vi "Code_rijden.vi"() -> ()   [LabVIEW 2014]
uses:
  <vilib>/LabVIEW Interface for Arduino/Type Defs/Board Type.ctl
  <vilib>/LabVIEW Interface for Arduino/Type Defs/Connection Type.ctl
  <vilib>/LabVIEW Interface for Arduino/LabVIEW Interface for Arduino.lvlib
panel:
  in  "Value (0)":u8
  in  "Banden Rechts":u8
  in  "Banden Links":u8
  in  "Achter Rechts":u8(slide) scale=0.0..255.0
  in  "Achter Links":u8(slide) scale=0.0..255.0
  in  "Voor Rechts":u8(slide) scale=0.0..255.0
  in  "Voor Links":u8(slide) scale=0.0..255.0
  in  "STOP":bool
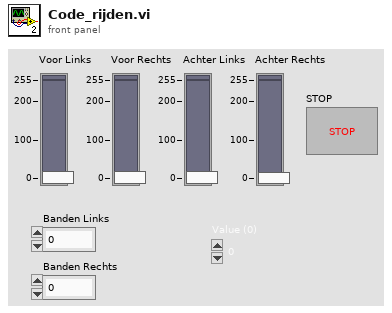
[diagram p1: front panel]
types:
  T1 = typedef "LabVIEW Interface for Arduino.lvlib/Connection Type.ctl" = enum8{"USB / Serial", "XBEE", "BlueSmirf (Bluetooth)"}
  T2 = typedef "LabVIEW Interface for Arduino.lvlib/Board Type.ctl" = enum16{"Uno", "Dimuelanove w/Atmega 328", "Mega 2560"}
  T3 = typedef "LabVIEW Interface for Arduino.lvlib/Arduino Resource.ctl" = cluster{"VISA resource":refnum<visa-resource-name>, "Board Type":T2, "Connection Type":enum8{"USB / Serial"}, "Bytes Per Packet (15)":u8}
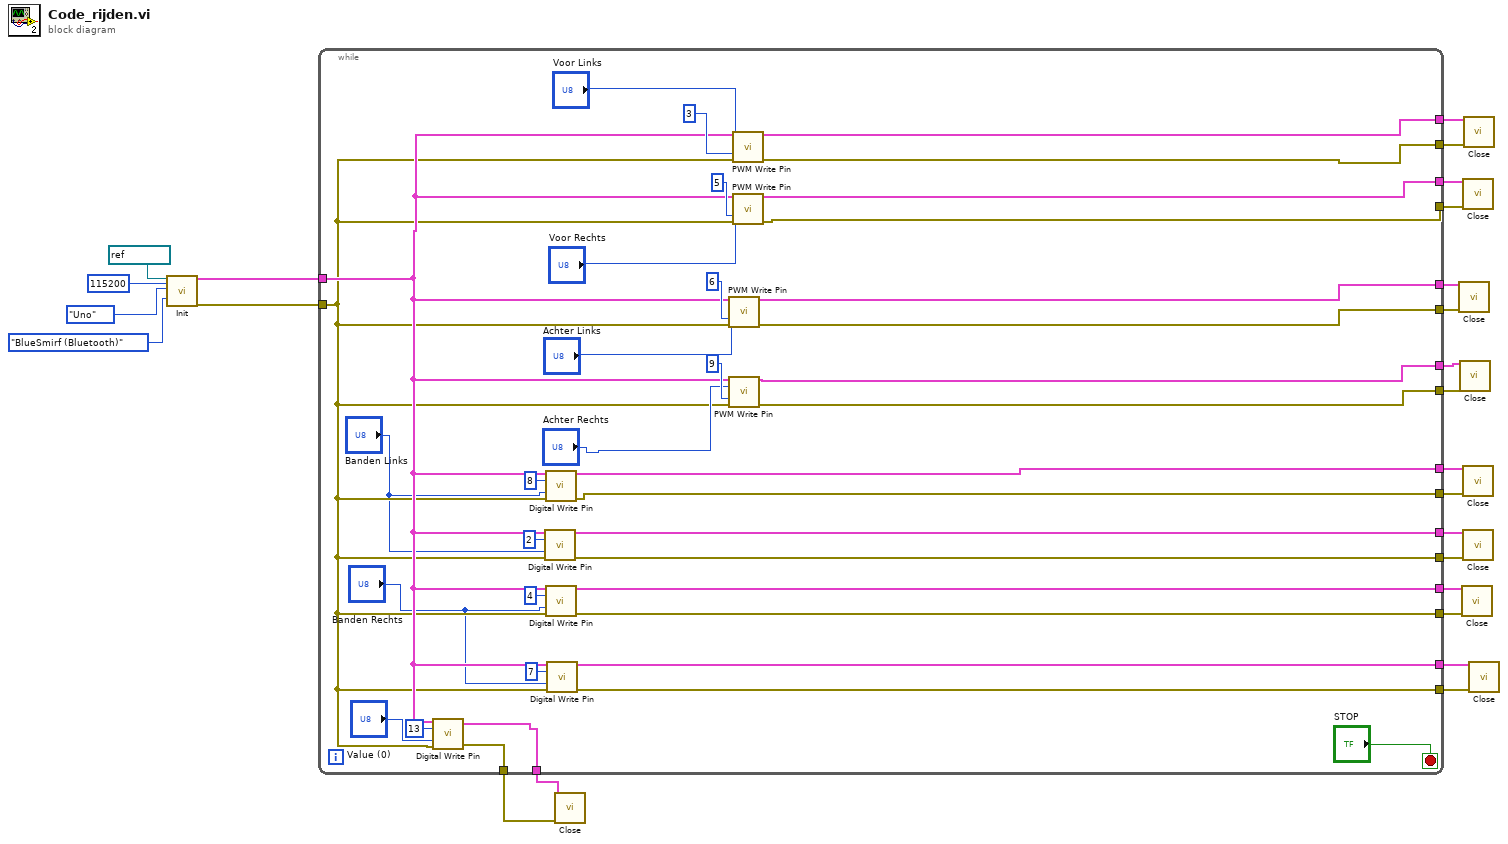
[diagram p0: block diagram]
diagram:
  n1 = call <vilib>:"Init.vi"("VISA resource"=refnum<visa-resource-name> "COM3", "Baud Rate (115200)"=u32 115200, "Board Type (Uno)"=Board_Type."Uno", "Connection Type (USB/Serial)"=Connection_Type."BlueSmirf (Bluetooth)") -> ("Arduino Resource"=w24:T3, "error out"=w23:errorcluster)  [unwired: 14 in]
  n2 = while {
    tunnel: w24 -> [w32]
    tunnel: w23 -> [w31]
    tunnel: [w56] -> w18
    tunnel: [w55] -> w17
    tunnel: [w54] -> w16
    tunnel: [w52] -> w15
    tunnel: [w51] -> w14
    tunnel: [w50] -> w13
    tunnel: [w49] -> w12
    tunnel: [w53] -> w11
    tunnel: [w44] -> w10
    tunnel: [w43] -> w9
    tunnel: [w42] -> w8
    tunnel: [w41] -> w7
    tunnel: [w40] -> w6
    tunnel: [w39] -> w5
    tunnel: [w38] -> w4
    tunnel: [w33] -> w3
    tunnel: [w28] -> w2
    tunnel: [w27] -> w1
    stop <- "STOP" stop-if-true
    n3 = call <vilib>:"Digital Write Pin.vi"("Arduino Resource"=w32, "Digital I/O Pin (0)"=u8 13, "Value (0)"="Value (0)", "error in"=w31) -> ("Arduino Resource"=w27:T3, "error out"=w28:errorcluster)  [unwired: 10 in]
    n4 = call <vilib>:"Digital Write Pin.vi"("Arduino Resource"=w32, "Digital I/O Pin (0)"=u8 2, "Value (0)"="Banden Links", "error in"=w31) -> ("Arduino Resource"=w40:T3, "error out"=w41:errorcluster)  [unwired: 10 in]
    n5 = call <vilib>:"Digital Write Pin.vi"("Arduino Resource"=w32, "Digital I/O Pin (0)"=u8 8, "Value (0)"="Banden Links", "error in"=w31) -> ("Arduino Resource"=w39:T3, "error out"=w38:errorcluster)  [unwired: 10 in]
    n6 = call <vilib>:"Digital Write Pin.vi"("Arduino Resource"=w32, "Digital I/O Pin (0)"=u8 4, "Value (0)"="Banden Rechts", "error in"=w31) -> ("Arduino Resource"=w33:T3, "error out"=w42:errorcluster)  [unwired: 10 in]
    n7 = call <vilib>:"Digital Write Pin.vi"("Arduino Resource"=w32, "Digital I/O Pin (0)"=u8 7, "Value (0)"="Banden Rechts", "error in"=w31) -> ("Arduino Resource"=w43:T3, "error out"=w44:errorcluster)  [unwired: 10 in]
    n8 = call <vilib>:"PWM Write Pin.vi"("Arduino Resource"=w32, "Duty Cycle (0 - 255)"="Achter Links", "PWM Pin (3)"=u8 6, "error in"=w31) -> ("Arduino Resource"=w52:T3, "error out"=w51:errorcluster)  [unwired: 10 in]
    n9 = call <vilib>:"PWM Write Pin.vi"("Arduino Resource"=w32, "Duty Cycle (0 - 255)"="Achter Rechts", "PWM Pin (3)"=u8 9, "error in"=w31) -> ("Arduino Resource"=w50:T3, "error out"=w49:errorcluster)  [unwired: 10 in]
    n10 = call <vilib>:"PWM Write Pin.vi"("Arduino Resource"=w32, "Duty Cycle (0 - 255)"="Voor Links", "PWM Pin (3)"=u8 3, "error in"=w31) -> ("Arduino Resource"=w56:T3, "error out"=w55:errorcluster)  [unwired: 10 in]
    n11 = call <vilib>:"PWM Write Pin.vi"("Arduino Resource"=w32, "Duty Cycle (0 - 255)"="Voor Rechts", "PWM Pin (3)"=u8 5, "error in"=w31) -> ("Arduino Resource"=w54:T3, "error out"=w53:errorcluster)  [unwired: 10 in]
  }
  n12 = call <vilib>:"Close.vi"("Arduino Resource"=w1, "error in"=w2) -> ()  [unwired: 13 in, 1 out]
  n13 = call <vilib>:"Close.vi"("Arduino Resource"=w15, "error in"=w14) -> ()  [unwired: 13 in, 1 out]
  n14 = call <vilib>:"Close.vi"("Arduino Resource"=w13, "error in"=w12) -> ()  [unwired: 13 in, 1 out]
  n15 = call <vilib>:"Close.vi"("Arduino Resource"=w3, "error in"=w8) -> ()  [unwired: 13 in, 1 out]
  n16 = call <vilib>:"Close.vi"("Arduino Resource"=w16, "error in"=w11) -> ()  [unwired: 13 in, 1 out]
  n17 = call <vilib>:"Close.vi"("Arduino Resource"=w5, "error in"=w4) -> ()  [unwired: 13 in, 1 out]
  n18 = call <vilib>:"Close.vi"("Arduino Resource"=w6, "error in"=w7) -> ()  [unwired: 13 in, 1 out]
  n19 = call <vilib>:"Close.vi"("Arduino Resource"=w18, "error in"=w17) -> ()  [unwired: 13 in, 1 out]
  n20 = call <vilib>:"Close.vi"("Arduino Resource"=w9, "error in"=w10) -> ()  [unwired: 13 in, 1 out]
